vi "test conversion.vi"() -> ()   [LabVIEW 2013, in "Profibus Module tests.lvlib"]
uses:
  Profibus Module tests.lvlib
  dynamic profibus/profibus master action.ctl
  dynamic profibus/full command.ctl
  dynamic profibus/dynamic profibus.lvlib
panel:
  out "ok? 2":bool
  in  "data 2":u8
  out "ok?":bool
  out "Element":u32
  in  "action":T1
  in  "device":u8
  in  "index":u8
  in  "data":u8
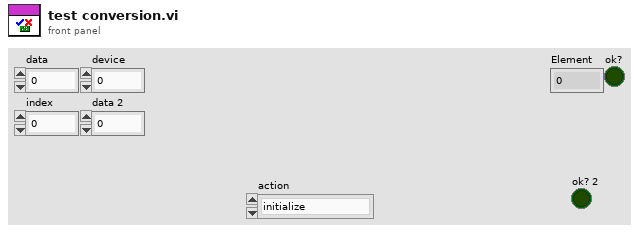
[diagram p1: front panel]
types:
  T1 = typedef "dynamic profibus.lvlib/profibus master action.ctl" = enum8{"initialize", "uninitialize", "stop", "get input", "get input size", "set output", "get output size", "get diagnostic", "transfer data", "transfer diagnostics", "read many inputs"}
  T2 = typedef "dynamic profibus.lvlib/full command.ctl" = cluster{"action":T1, "device":u8, "index":u8, "data":u8}
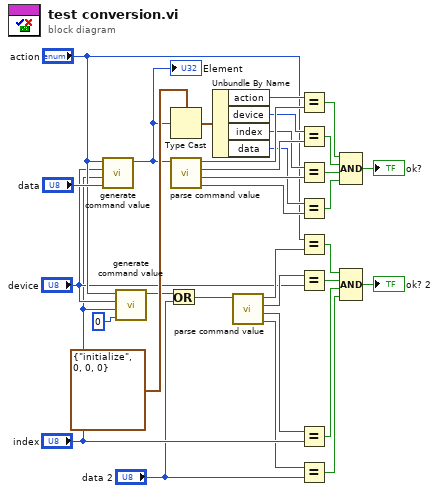
[diagram p0: block diagram]
diagram:
  n1 = call "generate command value.vi"("data"="data", "index"="index", "device"="device", "action"="action") -> ("Element"=w29:u32)  [unwired: 7 in]
  "Element" <- w29
  n2 = call "generate command value.vi"("data"=u8 0, "index"="index", "device"="device", "action"="action") -> ("Element"=w16:u32)  [unwired: 7 in]
  n3 = Or(x=w16, y="data 2") -> (x .or. y?=w14:u32)
  n4 = Type Cast(type=T2 {"action"=enum."initialize", "device"=0, "index"=0, "data"=0} ("command"), x=w29) -> (*(type *) &x=w31:T2)
  n5 = call "parse command value.vi"("Element"=w29) -> ("data"=w25:u8, "index"=w26:u8, "device"=w27:u8, "action"=w28:T1)  [unwired: 6 in, 1 out]
  n6 = Unbundle By Name(w31) -> ("action"=w30:T1, "device"=w24:u8, "index"=w23:u8, "data"=w22:u8)
  n7 = call "parse command value.vi"("Element"=w14) -> ("data"=w7:u8, "index"=w9:u8, "device"=w11:u8, "action"=w13:T1)  [unwired: 6 in, 1 out]
  n8 = Equal?(x=w30, y=w28) -> (x = y?=w18:bool)
  n9 = Equal?(x=w24, y=w27) -> (x = y?=w19:bool)
  n10 = Equal?(x=w23, y=w26) -> (x = y?=w20:bool)
  n11 = Equal?(x=w22, y=w25) -> (x = y?=w21:bool)
  n12 = Equal?(x="action", y=w13) -> (x = y?=w1:bool)
  n13 = Equal?(x=w11, y="device") -> (x = y?=w2:bool)
  n14 = Equal?(x=w9, y="index") -> (x = y?=w3:bool)
  n15 = Equal?(x=w7, y="data 2") -> (x = y?=w4:bool)
  n16 = Compound Arithmetic op=AND(w18, w19, w20, w21) -> (→"ok?":bool)
  n17 = Compound Arithmetic op=AND(w1, w2, w3, w4) -> (→"ok? 2":bool)
